vi "Grid KeyDown.vi"(8 "error in (no error)":errorcluster caption="エラー入力（エラーなし）", 9 "VKey":T3, 10 "Char":i16, 11 "表関係クラスタ":T4) -> (0 "error out":errorcluster caption="エラー出力", 3 "破棄?":bool)   [LabVIEW 2014]
uses:
  <vilib>/event_ctls.llb/eventvkey.ctl
  Grid Parameter.ctl
  <vilib>/Utility/miscctls.llb/LVPositionTypeDef.ctl
  <vilib>/Utility/miscctls.llb/LVRowAndColumnTypeDef.ctl
panel:
  out "編集位置":T1
  out "アクティブセル:位置":T2
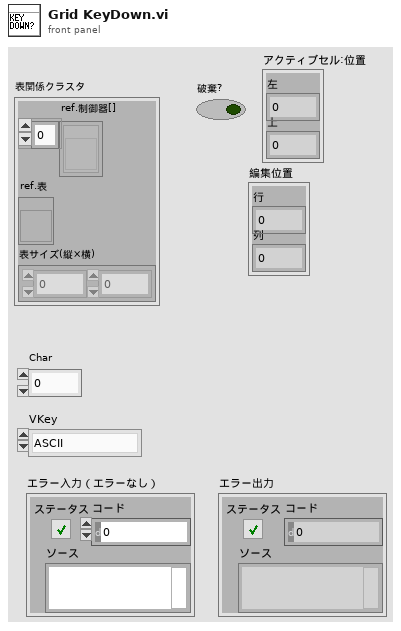
[diagram p1: front panel]
types:
  T1 = typedef "LVRowAndColumnTypeDef.ctl" = cluster{"Row":i32, "Column":i32}
  T2 = typedef "LVPositionTypeDef.ctl" = cluster{"Left":i32, "Top":i32}
  T3 = typedef "eventvkey.ctl" = enum16{"ASCII", "Enter", "Return", "Shift", "Ctrl", "Alt", "Cmd", "Opt", "Caps", "NumLock", "Clear", "Break", "Up", "Down", "Left", "Right", "Insert", "Delete", "Home", "End", "PageUp", "PageDown", "Escape", "Help", "Pause", "ScrollLock", "F1", "F2", "F3", "F4", "F5", "F6", "F7", "F8", "F9", "F10", "F11", "F12", "F13", "F14", "F15", "F16", "F17", "F18", "F19", "F20", "F21", "F22", "F23", "F24", "Play", "VolumeUp", "VolumeDown", "Mute", "Two Byte Char"}
  T4 = typedef "Grid Parameter.ctl" = cluster{"ref.制御器[]":refnum<vi>[], "ref.表":refnum<vi>, "表サイズ(縦×横)":i32[]}
  T5 = typedef "Clust ClassID.ctl" = enum16{"０", "１", "２", "３", "４", "５", "６", "色", "ブール", "９", "１０", "パス", "１２", "１３", "配列", "１５", "１６", "１７", "数値", "１９", "２０", "２１", "２２", "２３", "２４", "２５", "２６", "文字列", "２８", "２９", "３０", "３１", "３２", "３３", "リング", "Enum", "３６"}
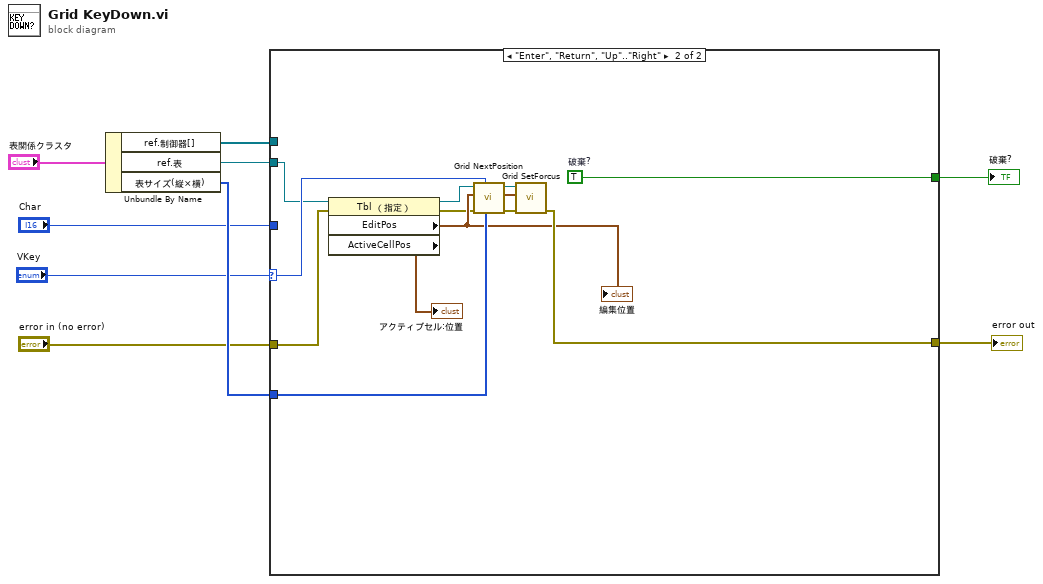
[diagram p0: block diagram]
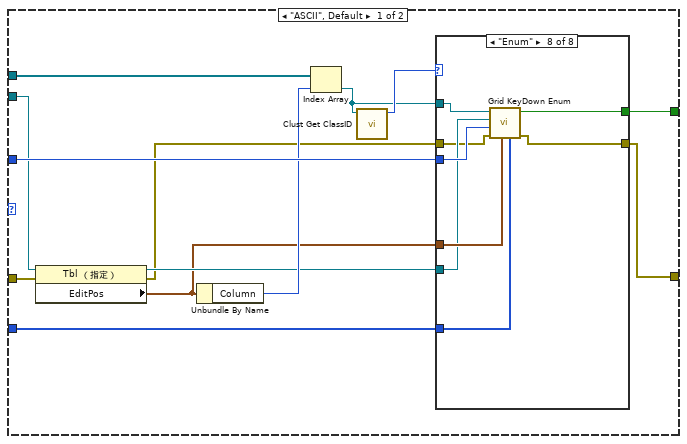
[diagram p2: hidden frame]
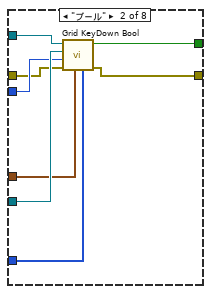
[diagram p4: hidden frame]
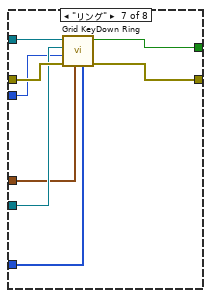
[diagram p9: hidden frame]
diagram:
  n1 = Unbundle By Name("表関係クラスタ") -> ("ref.制御器[]"=w8:refnum<vi>[], "ref.表"=w3:refnum<vi>, "表サイズ(縦×横)"=w9:i32[])
  n2 = case shown="\"Enter\", \"Return\", \"Up\"..\"Right\"" "VKey" {
    selector: "VKey" -> [_ w59]
    tunnel: "Char" -> [w21 _]
    tunnel: [w22 w64] -> w4
    tunnel: w8 -> [w10 _]
    tunnel: w9 -> [w18 w63]
    tunnel: w3 -> [w16 w57]
    tunnel: "error in (no error)" -> [w13 w53]
    tunnel: [w12 w58] -> w1
    frame "ASCII", Default {
      n3 = property class="Tbl （指定）"(reference=w16, error in=w13) -> (reference out=w15:refnum<vi>, error out=w11:errorcluster, "EditPos"=w14:T1)
      n4 = Unbundle By Name(w14) -> ("Column"=w20:i32)
      n5 = Index Array(array=w10, index=w20) -> (element=w17:refnum<vi>)
      n6 = call "Clust Get ClassID.vi"("Ctl Refnum"=w17) -> ("ClassID"=w19:T5)  [unwired: 10 in]
      n7 = case shown="\"Enum\"" w19 {
        tunnel: w21 -> [_ w28 _ _ _ _ w39 w51]
        tunnel: w14 -> [_ w29 _ _ _ _ w38 w49]
        tunnel: [_ w27 _ _ _ _ w42 w48] -> w22
        tunnel: w17 -> [_ w31 _ _ _ _ w43 w50]
        tunnel: w18 -> [_ w26 _ _ _ _ w37 w46]
        tunnel: w15 -> [_ w30 _ _ _ _ w40 w47]
        tunnel: w11 -> [w23 w25 w32 w33 w34 w35 w41 w45]
        tunnel: [w23 w24 w32 w33 w34 w35 w36 w44] -> w12
        frame Default {
        }
        frame "ブール" {
          n8 = call "Grid KeyDown Bool.vi"("表サイズ(縦×横)"=w26, "EditPos"=w29, "error in (no error)"=w25, "Char"=w28, "ref.表"=w30, "Control入力"=w31) -> ("error out"=w24:errorcluster, "ブール"=w27:bool)  [unwired: 3 in, 1 out]
        }
        frame "パス" {
        }
        frame "配列" {
        }
        frame "数値" {
        }
        frame "文字列" {
        }
        frame "リング" {
          n9 = call "Grid KeyDown Ring.vi"("表サイズ(縦×横)"=w37, "EditPos"=w38, "エラー入力（エラーなし）"=w41, "Char"=w39, "ref.表"=w40, "Control入力"=w43) -> ("error out"=w36:errorcluster, "破棄?"=w42:bool)  [unwired: 3 in, 1 out]
        }
        frame "Enum" {
          n10 = call "Grid KeyDown Enum.vi"("表サイズ(縦×横)"=w46, "EditPos"=w49, "error in (no error)"=w45, "Char"=w51, "ref.表"=w47, "Control入力"=w50) -> ("error out"=w44:errorcluster, "ブール"=w48:bool)  [unwired: 3 in, 1 out]
        }
      }
    }
    frame "Enter", "Return", "Up".."Right" {
      w64 = TRUE  # 破棄?
      n11 = property class="Tbl （指定）"(reference=w57, error in=w53) -> (reference out=w54:refnum<vi>, error out=w55:errorcluster, "EditPos"=w56:T1, "ActiveCellPos"=→"アクティブセル:位置":T2)
      "編集位置" <- w56
      n12 = call "Grid NextPosition.vi"("表サイズ(縦x横)"=w63, "VKey(Right)"=w59, "error in (no error)"=w55, "EditPos入力"=w56, "ref.表"=w54) -> ("error out"=w61:errorcluster, "EditPos出力"=w60:T1, "ref.表(copy)"=w62:refnum<vi>)  [unwired: 4 in]
      n13 = call "Grid SetForcus.vi"("エラー入力（エラーなし）"=w61, "EditPos入力"=w60, "Table入力"=w62) -> ("error out"=w58:errorcluster)  [unwired: 6 in, 2 out]
    }
  }
  "破棄?" <- w4
  "error out" <- w1
